vi "User Interface.vi"(8 "error in (no error)":errorcluster, 11 "User Interface in":refnum<class "User Interface.lvclass">) -> (0 "error out":errorcluster, 3 "User Interface in":refnum<class "User Interface.lvclass">)   [LabVIEW 2017, in "DSF Core.lvlib" / "Core Plugin User Interface.lvclass"]
uses:
  Core Plugin User Interface.lvclass
  User Interface.lvclass
  Configuration/Base/Plugin/Plugin Configuration.lvclass
  C:/Git/DSF/Core/Classes/Configuration/Configuration.lvclass
  Configuration/Configuration.lvclass
panel:
  in  "Offset":u64
  in  "Decimation":u64
  in  "Priority":u64
  in  "Components":string[](array[string])
  in  "Name":string
  out "Data Version":string
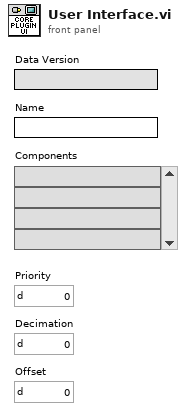
[diagram p1: front panel]
types:
  T1 = typedef "DSF Core.lvlib/DSF Core Plugin Configuration.ctl" = cluster{"name":string, "components":string[], "cycle timing":T2}
  T2 = typedef "DSF Core.lvlib/DSF Timing Info.ctl" = cluster{"priority":u64, "decimation":u64, "offset":u64}
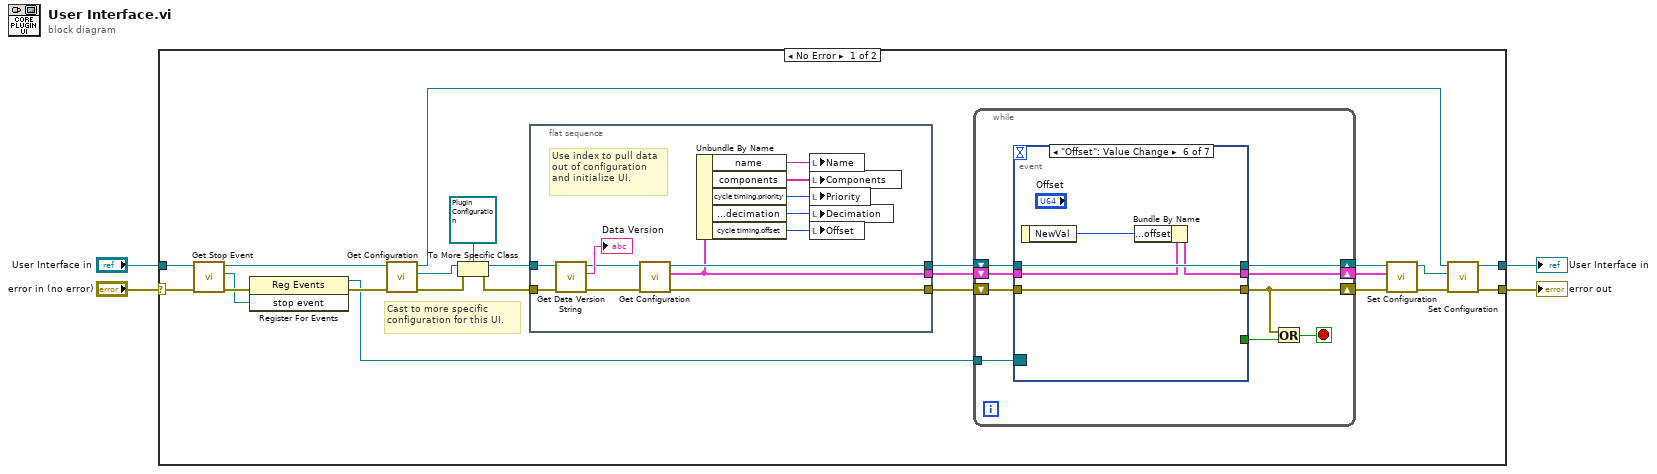
[diagram p0: block diagram]
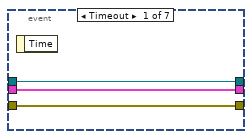
[diagram p2: hidden frame]
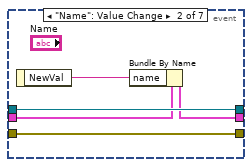
[diagram p3: hidden frame]
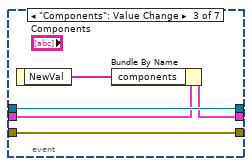
[diagram p4: hidden frame]
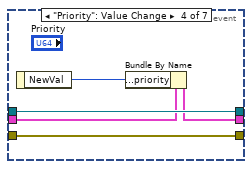
[diagram p5: hidden frame]
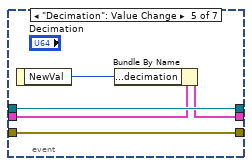
[diagram p6: hidden frame]
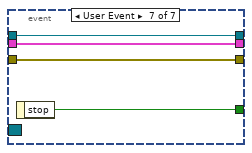
[diagram p7: hidden frame]
diagram:
  n1 = case shown="No Error" "error in (no error)" {
    selector: "error in (no error)" -> [w21 w83]
    tunnel: [w12 w83] -> w4
    tunnel: "User Interface in" -> [w20 w82]
    tunnel: [w13 w82] -> w1
    frame No Error {
      # "Cast to more specific configuration for this UI."
      n2 = call "Get Stop Event.vi"("error in (no error)"=w21, "User Interface in"=w20) -> ("error out"=w19:errorcluster, "stop event"=w18:refnum<user-event>, "User Interface out"=w22:refnum<class "User Interface.lvclass">)  [unwired: 7 in]
      n3 = register-events(error in=w19, w18) -> (reference out=w11:refnum<event-registration>, error out=w17:errorcluster)  [unwired: 1 in]
      n4 = call "Get Configuration.vi"("error in (no error)"=w17, "User Interface in"=w22) -> ("error out"=w16:errorcluster, "configuration"=w15:refnum<class "Configuration.lvclass">, "User Interface out"=w14:refnum<class "User Interface.lvclass">)  [unwired: 7 in]
      n5 = To More Specific Class(target class=refnum<class "Plugin Configuration.lvclass"> refnum ("DSF Core.lvlib:Plugin Configuration.lvclass"), reference=w15, error in=w16) -> (specific class reference=w27:refnum<class "Plugin Configuration.lvclass">, error out=w24:errorcluster)
      n6 = flat-sequence {
        tunnel: [w29] -> w25
        tunnel: w24 -> [w40]
        tunnel: w27 -> [w39]
        tunnel: [w30] -> w26
        tunnel: [w28] -> w23
        frame #0 {
          # "Use index to pull data out of configuration and initialize UI."
          n7 = call "Get Data Version String.vi"("error in (no error)"=w40, "Configuration in"=w39) -> ("error out"=w32:errorcluster, "data version"=→"Data Version":string, "Configuration out"=w31:refnum<class "Plugin Configuration.lvclass">)  [unwired: 7 in]
          n8 = call "Get Configuration.vi"("error in (no error)"=w32, "Core Plugins Configuration in"=w31) -> ("error out"=w29:errorcluster, "configuration"=w28:T1, "Core Plugins Configuration out"=w30:refnum<class "Plugin Configuration.lvclass">)  [unwired: 7 in]
          n9 = Unbundle By Name(w28) -> ("name"=w37:string, "components"=w36:string[], "cycle timing.priority"=w35:u64, "cycle timing.decimation"=w34:u64, "cycle timing.offset"=w33:u64)
          n10 = local write "Name"(w37) -> ()
          n11 = local write "Components"(w36) -> ()
          n12 = local write "Priority"(w35) -> ()
          n13 = local write "Decimation"(w34) -> ()
          n14 = local write "Offset"(w33) -> ()
        }
      }
      n15 = while {
        tunnel: w11 -> [w49]
        shift-right: [w47] -> w9
        shift-left: w25 -> [w48]
        shift-right: [w43] -> w7
        shift-left: w26 -> [w44]
        shift-right: [w41] -> w5
        shift-left: w23 -> [w42]
        stop <- w46 stop-if-true
        n16 = event shown="[5] \"Offset\": Value Change" {
          selector: w49 -> [_ _ _ _ _ _ _]
          dyn-events: _ -> [_ _ _ _ _ _ _]
          timeout: _ -> [_ _ _ _ _ _ _]
          tunnel: [_ _ _ _ _ _ w79] -> w45
          tunnel: w48 -> [w52 w57 w62 w67 w72 w77 w81]
          tunnel: [w52 w57 w62 w67 w72 w77 w81] -> w47
          tunnel: w44 -> [w51 w56 w61 w66 w71 w76 w80]
          tunnel: [w51 w56 w61 w66 w71 w76 w80] -> w43
          tunnel: w42 -> [w50 w55 w60 w65 w70 w75 w78]
          tunnel: [w50 w54 w59 w64 w69 w74 w78] -> w41
          event Timeout {
            n17 = event-data() -> ()  [unwired: 1 in, 1 out]
          }
          event "Name": Value Change {
            n18 = event-data() -> ("NewVal"=w53:string)  [unwired: 1 in]
            n19 = Bundle By Name(cluster=w55, "name"=w53) -> (w54:T1)
          }
          event "Components": Value Change {
            n20 = event-data() -> ("NewVal"=w58:string[])  [unwired: 1 in]
            n21 = Bundle By Name(cluster=w60, "components"=w58) -> (w59:T1)
          }
          event "Priority": Value Change {
            n22 = event-data() -> ("NewVal"=w63:u64)  [unwired: 1 in]
            n23 = Bundle By Name(cluster=w65, "cycle timing.priority"=w63) -> (w64:T1)
          }
          event "Decimation": Value Change {
            n24 = event-data() -> ("NewVal"=w68:u64)  [unwired: 1 in]
            n25 = Bundle By Name(cluster=w70, "cycle timing.decimation"=w68) -> (w69:T1)
          }
          event "Offset": Value Change {
            n26 = event-data() -> ("NewVal"=w73:u64)  [unwired: 1 in]
            n27 = Bundle By Name(cluster=w75, "cycle timing.offset"=w73) -> (w74:T1)
          }
          event User Event {
            n28 = event-data() -> ("stop"=w79:bool)  [unwired: 1 in]
          }
        }
        n29 = Or(x=w47, y=w45) -> (x .or. y?=w46:bool)
      }
      n30 = call "Set Configuration.vi"("error in (no error)"=w9, "configuration"=w5, "Core Plugins Configuration in"=w7) -> ("error out"=w8:errorcluster, "Core Plugins Configuration out"=w6:refnum<class "Plugin Configuration.lvclass">)  [unwired: 7 in]
      n31 = call "Set Configuration.vi"("error in (no error)"=w8, "configuration"=w6, "User Interface in"=w14) -> ("error out"=w12:errorcluster, "User Interface out"=w13:refnum<class "User Interface.lvclass">)  [unwired: 7 in]
    }
    frame Error {
    }
  }
  "error out" <- w4
  "User Interface in" <- w1
